vi "Core Cleanup.vi"(8 "error in (no error)":errorcluster, 11 "CIFTemplateNode in":refnum<class "CIFCorePlugin.lvclass">) -> (0 "error out":errorcluster, 3 "CIFTemplateNode out":refnum<class "CIFCorePlugin.lvclass">)   [LabVIEW 2021, in "CIFCorePlugin.lvclass"]
uses:
  CIFCorePlugin.lvclass
  CIFCorePlugin.lvclass/CIFCorePlugin.ctl
  Typedef/Energized States.ctl
  Common/Typedef/Plugin State.ctl
  <vilib>/CIF Foundation/CIF Utilities/Statistics/I64/Stats_I64_CIF_U.lvclass/Stats_I64_CIF_U.ctl
  <vilib>/CIF Foundation/CIF Utilities/Time/System Time/Get System Time.vi
  <vilib>/CIF Foundation/CIF Utilities/Statistics/I64/X1 minus X0.vi
  Accessors/Timestamps/Read Cleanup TS.vi
  <vilib>/CIF Foundation/CIF Utilities/Statistics/I64/X1 minus X0.vi/dfabcf33-0dbc-4041-80a5-3dc0c86d2989.vi
  <vilib>/CIF Foundation/CIF Utilities/Statistics/I64/X1 minus X0.vi/dfabcf33-0dbc-4041-80a5-3dc0c86d2989.vi/9eb60a9a-770f-4d2d-8b3f-8465c267ecc9.vi
  Logs/Log State Change.vi
  Common/CIFCoreCommon.lvlib
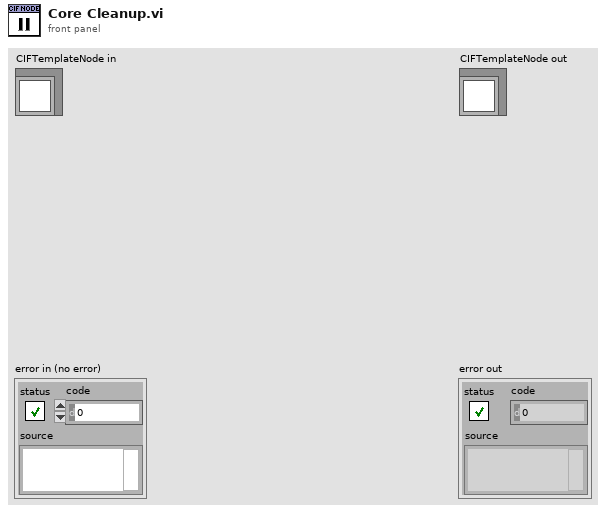
[diagram p1: front panel]
types:
  T1 = typedef "CIFCorePlugin.lvclass/Energized States.ctl" = enum8{"Listen", "Prepare", "Execute", "Housekeep", "Cleanup", "Destroy"}
  T2 = typedef "CIFCoreCommon.lvlib/Plugin State.ctl" = enum8{"Null", "Creating", "Listening", "Running", "CleaningUp", "Destroying", "Prepared", "FTE_Run"}
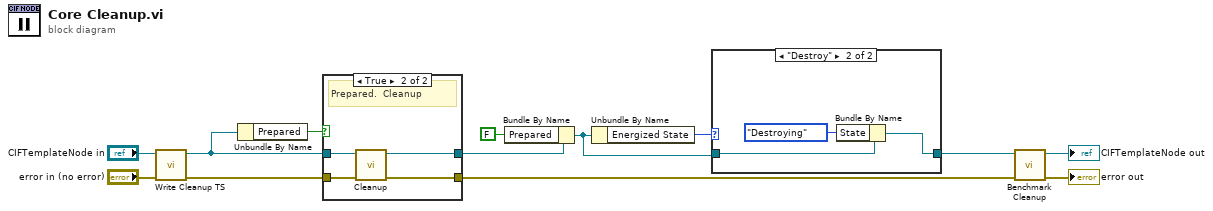
[diagram p0: block diagram]
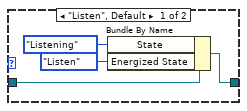
[diagram p3: hidden frame]
diagram:
  n1 = call "Write Cleanup TS.vi"("error in (no error)"="error in (no error)", "CIFCorePlugin in"="CIFTemplateNode in") -> ("error out"=w11:errorcluster, "CIFCorePlugin out"=w5:refnum<class "CIFCorePlugin.lvclass">)  [unwired: 8 in]
  n2 = Unbundle By Name(w5) -> ("Prepared"=w4:bool)
  n3 = case shown="True" w4 {
    tunnel: w11 -> [w14 w19]
    tunnel: [w15 w18] -> w3
    tunnel: [w14 w17] -> w8
    tunnel: w5 -> [w15 w16]
    frame False {
      # "Never prepared, skip cleanup"
    }
    frame True {
      # "Prepared.  Cleanup"
      n4 = call-dynamic "Cleanup.vi"("error in (no error)"=w19, "CIFTemplateNode in"=w16) -> ("error out"=w17:errorcluster, "CIFTemplateNode out"=w18:refnum<class "CIFCorePlugin.lvclass">)  [unwired: 8 in]
    }
  }
  n5 = Bundle By Name(cluster=w3, "Prepared"=FALSE ("Running Internal Data.Prepared")) -> (w2:refnum<class "CIFCorePlugin.lvclass">)
  n6 = Unbundle By Name(w2) -> ("Energized State"=w10:T1)
  n7 = case shown="\"Destroy\"" w10 {
    tunnel: w2 -> [w23 w26]
    tunnel: [w21 w25] -> w9
    frame "Listen", Default {
      n8 = Bundle By Name(cluster=w23, "State"=Plugin_State."Listening" ("Main to gRPC Data.Status.State"), "Energized State"=Energized_States."Listen") -> (w21:refnum<class "CIFCorePlugin.lvclass">)
    }
    frame "Destroy" {
      n9 = Bundle By Name(cluster=w26, "State"=Plugin_State."Destroying" ("Main to gRPC Data.Status.State")) -> (w25:refnum<class "CIFCorePlugin.lvclass">)
    }
  }
  n10 = call "Benchmark Cleanup.vi"("error in (no error)"=w8, "CIFCorePlugin in"=w9) -> ("error out"=→"error out":errorcluster, "CIFCorePlugin out"=→"CIFTemplateNode out":refnum<class "CIFCorePlugin.lvclass">)  [unwired: 8 in]
